vi "MouseScale.vi"(1 "NumMonitors":i32, 2 "ScreenCluster":T3={"Screen1"={"ScreenWidth"=1440.0, "ScreenHeight"=900.0}, "Screen2"={"ScreenWidth"=1440.0, "ScreenHeight"=900.0}} {"Screen2"."ScreenHeight" step=0.5; "Screen1"."ScreenHeight" step=0.5}, 3 "button info":T1, 4 "axis info":T4) -> (0 "MouseCluster":T2)   [LabVIEW 2010]
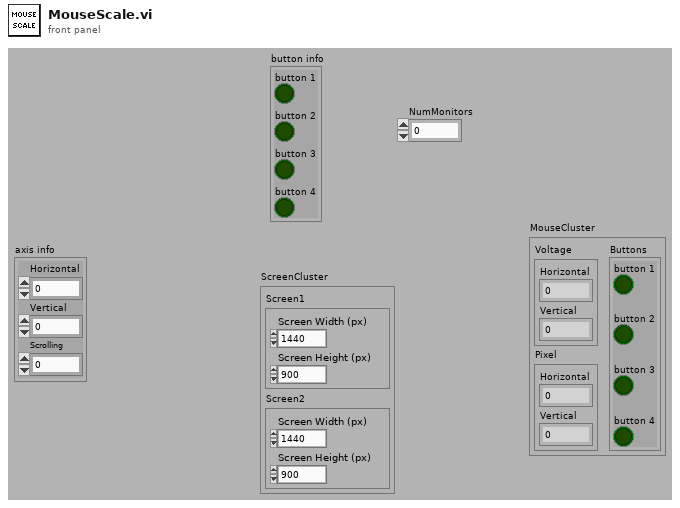
[diagram p1: front panel]
types:
  T1 = cluster{"button 1":bool, "button 2":bool, "button 3":bool, "button 4":bool}
  T2 = cluster{"Voltage":cluster{"Horizontal":dbl, "Vertical":dbl}, "Pixel":cluster{"Horizontal":dbl, "Vertical":dbl}, "Buttons":cluster{"button 1":bool, "button 2":bool, "button 3":bool, "button 4":bool}}
  T3 = cluster{"Screen1":cluster{"ScreenWidth":dbl, "ScreenHeight":dbl}, "Screen2":cluster{"ScreenWidth":dbl, "ScreenHeight":dbl}}
  T4 = cluster{"Horizontal":i32, "Vertical":i32, "Scrolling":i32}
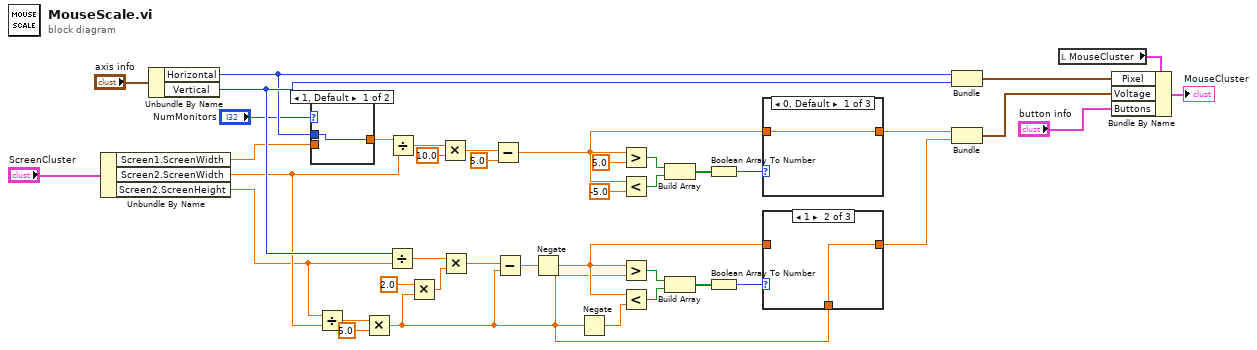
[diagram p0: block diagram]
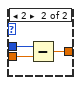
[diagram p2: hidden frame]
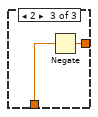
[diagram p4: hidden frame]
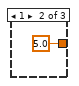
[diagram p5: hidden frame]
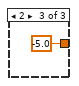
[diagram p6: hidden frame]
diagram:
  n1 = Unbundle By Name("ScreenCluster") -> ("Screen1.ScreenWidth"=w4:dbl, "Screen2.ScreenWidth"=w3:dbl, "Screen2.ScreenHeight"=w2:dbl)
  n2 = Unbundle By Name("axis info") -> ("Horizontal"=w5:i32, "Vertical"=w13:i32)
  n3 = case shown="1, Default" "NumMonitors" {
    tunnel: [w42 w45] -> w7
    tunnel: w5 -> [w42 w44]
    tunnel: w4 -> [_ w43]
    frame 1, Default {
    }
    frame 2 {
      n4 = Subtract(x=w44, y=w43) -> (x-y=w45:dbl)
    }
  }
  n5 = Divide(x=w2, y=w3) -> (x/y=w21:dbl)
  n6 = Multiply(x=w21, y=5.0) -> (x*y=w16:dbl)
  n7 = Divide(x=w13, y=w2) -> (x/y=w36:dbl)
  n8 = Divide(x=w7, y=w3) -> (x/y=w39:dbl)
  n9 = Multiply(x=2.0, y=w16) -> (x*y=w19:dbl)
  n10 = Multiply(x=w39, y=10.0) -> (x*y=w37:dbl)
  n11 = Multiply(x=w36, y=w19) -> (x*y=w35:dbl)
  n12 = Subtract(x=w37, y=5.0) -> (x-y=w27:dbl)
  n13 = Subtract(x=w35, y=w16) -> (x-y=w34:dbl)
  n14 = Negate(x=w34) -> (-x=w22:dbl)
  n15 = Negate(x=w16) -> (-x=w17:dbl)
  n16 = Greater?(x=w27, y=5.0) -> (0:w31:bool)
  n17 = Less?(x=w27, y=-5.0) -> (x < y?=w30:bool)
  n18 = Greater?(x=w22, y=w16) -> (0:w23:bool)
  n19 = Less?(x=w22, y=w17) -> (x < y?=w24:bool)
  n20 = Build Array(w31, w30) -> (w29:bool[])
  n21 = Build Array(w23, w24) -> (w25:bool[])
  n22 = Boolean Array To Number(Boolean array=w29) -> (number=w28:u32)
  n23 = Boolean Array To Number(Boolean array=w25) -> (number=w26:u32)
  n24 = case shown="0, Default" w28 {
    tunnel: w27 -> [w46 _ _]
    tunnel: [w46 5.0 -5.0] -> w11
    frame 0, Default {
    }
    frame 1 {
    }
    frame 2 {
    }
  }
  n25 = case shown="1" w26 {
    tunnel: w22 -> [w49 _ _]
    tunnel: [w49 w50 w52] -> w10
    tunnel: w16 -> [_ w50 w51]
    frame 0, Default {
    }
    frame 1 {
    }
    frame 2 {
      n26 = Negate(x=w51) -> (-x=w52:dbl)
    }
  }
  n27 = Bundle("Horizontal"=w5, "Vertical"=w13) -> (w12:cluster{"Horizontal":i32, "Vertical":i32})  [unwired: 1 in]
  n28 = Bundle(w11, w10) -> (w9:cluster{dbl, dbl})  [unwired: 1 in]
  n29 = local read "MouseCluster"() -> (w15:T2)
  n30 = Bundle By Name(cluster=w15, "Pixel"=w12, "Voltage"=w9, "Buttons"="button info") -> (→"MouseCluster":T2)
